vi "Random XY Generator.vi"(4 "Max h variatie":dbl=5.0, 5 "Max V variatie":dbl=1.0, 6 "Random Methode":u16(ring)=1 items=["Methode Random", "Methode smooth"], 7 "Y start":dbl=30.0, 8 "X start":dbl=61.0, 9 "number of rounds":i32=1) -> (0 "Array":cluster{"x":dbl, "y":dbl, "v":dbl, "h":dbl}[](array[cluster]), 1 "Array":dbl[][](array[numeric]), 2 "Y end randomized":dbl, 3 "X end randomized":dbl)   [LabVIEW 2014]
panel:
  out "XY Graph 2":cluster{dbl[], dbl[]}(graph)
  out "Y start 2":dbl
  out "X start 2":dbl
  out "Waveform Graph 2":dbl[](graph)
  out "Waveform Graph":dbl[](graph)
  out "XY Graph":cluster{dbl[], dbl[]}(graph)
  in  "Step Time [Sec]":dbl=1.0
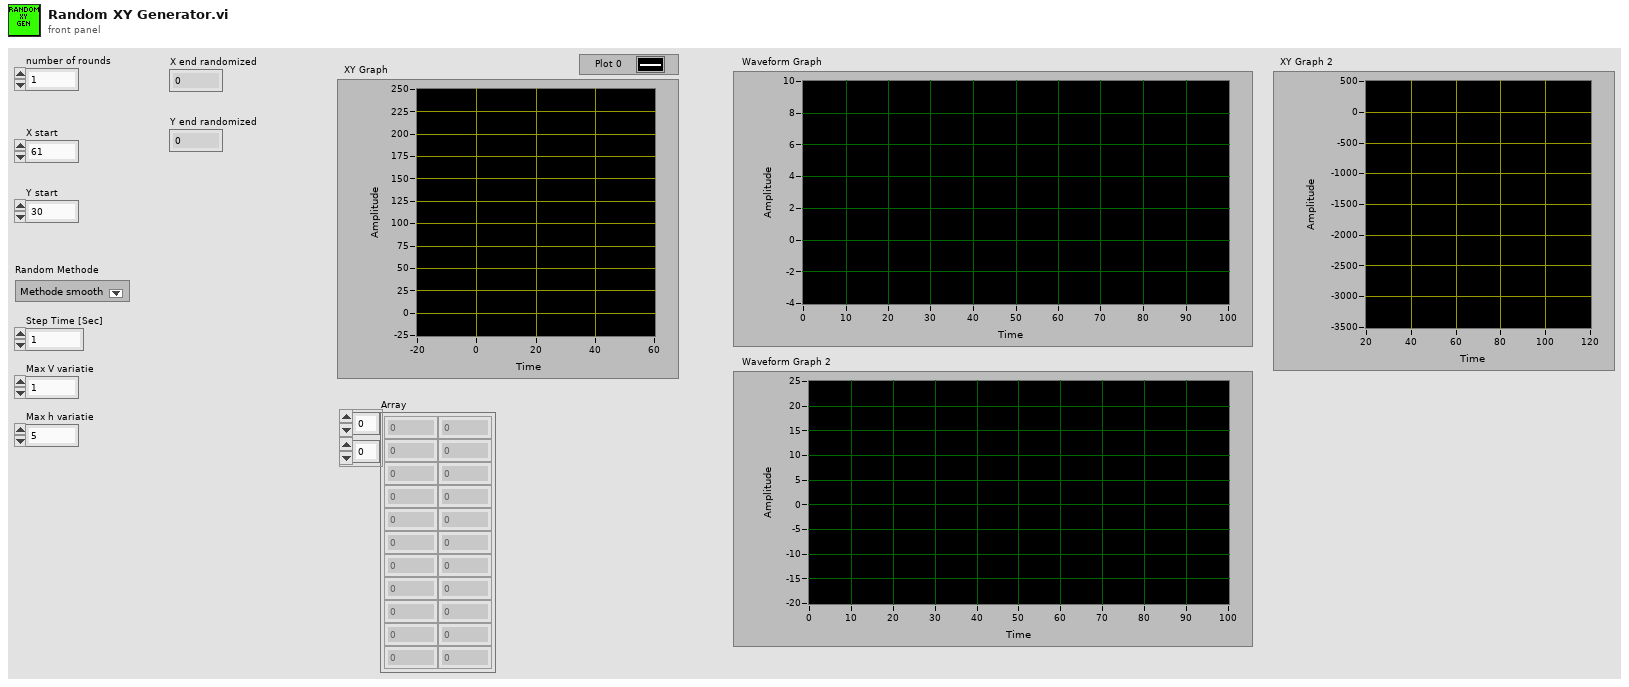
[diagram p1: front panel]
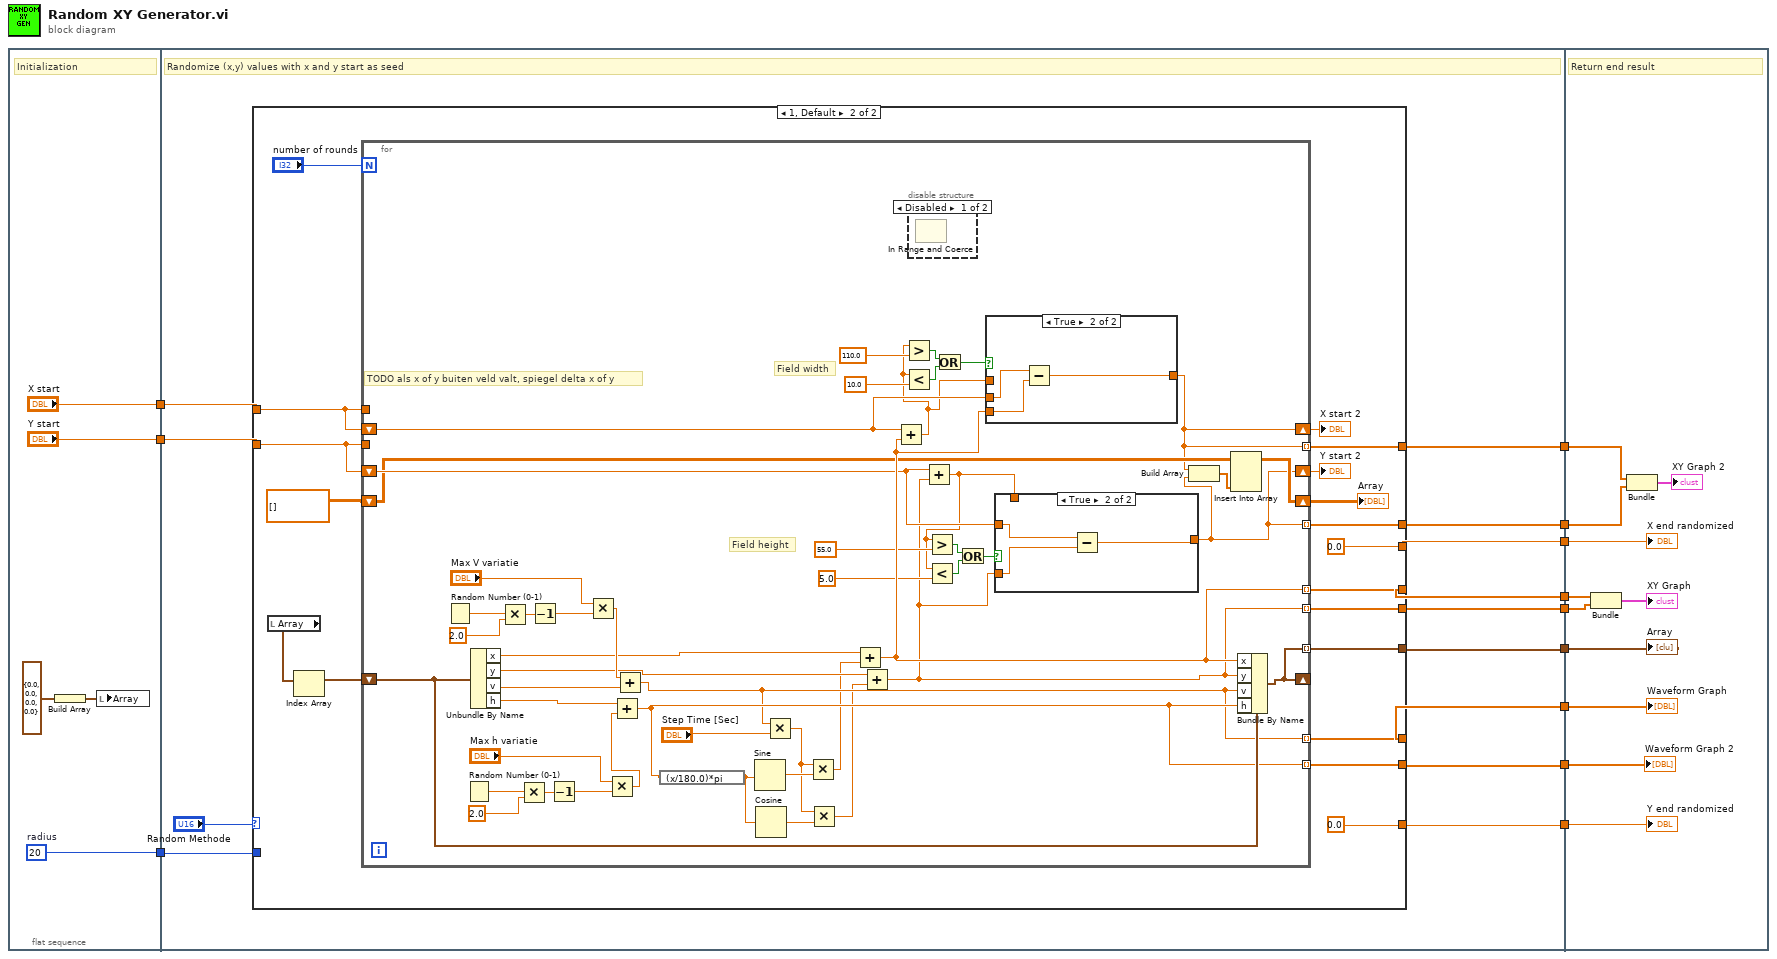
[diagram p0: block diagram]
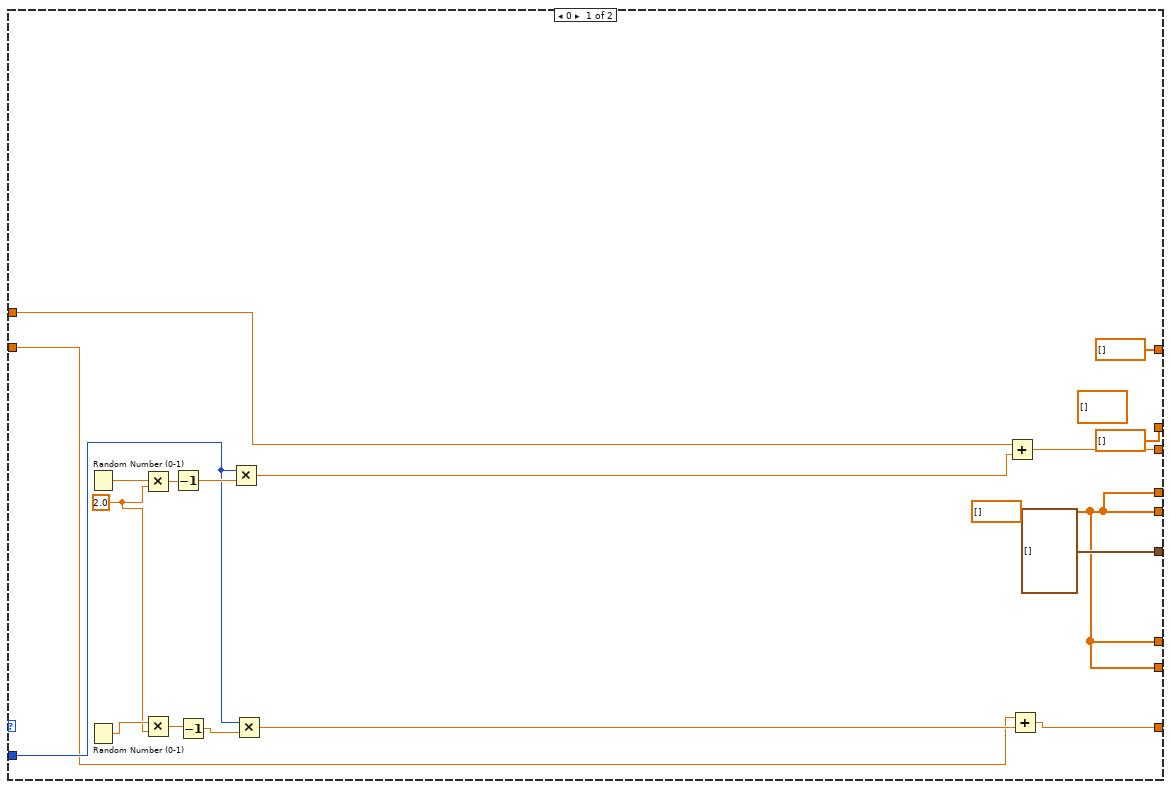
[diagram p2: hidden frame]
diagram:
  n1 = flat-sequence {
    tunnel: ["X start"] -> w12
    tunnel: ["Y start"] -> w11
    tunnel: [w15] -> w10
    tunnel: w12 -> [w29]
    tunnel: w11 -> [w28]
    tunnel: w10 -> [w30]
    tunnel: [w27] -> w9
    tunnel: [w26] -> w8
    tunnel: [w24] -> w7
    tunnel: [w23] -> w6
    tunnel: [w22] -> w5
    tunnel: [w21] -> w4
    tunnel: [w20] -> w3
    tunnel: [w19] -> w2
    tunnel: [w18] -> w1
    tunnel: w9 -> [w133]
    tunnel: w8 -> [w132]
    tunnel: w7 -> [w131]
    tunnel: w6 -> [w130]
    tunnel: w5 -> [w129]
    tunnel: w4 -> [w127]
    tunnel: w3 -> [w126]
    tunnel: w2 -> [w124]
    tunnel: w1 -> [w123]
    frame #0 {
      w15 = 20  # radius
      # "Initialization"
      n2 = Build Array(cluster{"x":dbl, "y":dbl, "v":dbl, "h":dbl} {"x"=0.0, "y"=0.0, "v"=0.0, "h"=0.0} ("Cluster")) -> (w13:cluster{"x":dbl, "y":dbl, "v":dbl, "h":dbl}[])
      n3 = local write "Array"(w13) -> ()
    }
    frame #1 {
      # "Randomize (x,y) values with x and y start as seed"
      n4 = case shown="1, Default" "Random Methode" {
        tunnel: w30 -> [w41 _]
        tunnel: w29 -> [w39 w57]
        tunnel: w28 -> [w37 w56]
        tunnel: [w36 0.0] -> w27
        tunnel: [w35 0.0] -> w26
        tunnel: [cluster{"x":dbl, "y":dbl, "v":dbl, "h":dbl}[] [] w66] -> w24
        tunnel: [w33 w63] -> w23
        tunnel: [w33 w62] -> w22
        tunnel: [w33 w59] -> w21
        tunnel: [w33 w58] -> w20
        tunnel: [dbl[] [] w51] -> w19
        tunnel: [dbl[] [] w50] -> w18
        frame 0 {
          (unwired) dbl[][] []
          w33 = dbl[] []
          w46 = 2.0
          n5 = Random Number (0-1)() -> (number: 0 to 1=w48:dbl)
          n6 = Random Number (0-1)() -> (number: 0 to 1=w47:dbl)
          n7 = Multiply(x=w48, y=w46) -> (x*y=w45:dbl)
          n8 = Multiply(x=w47, y=w46) -> (x*y=w44:dbl)
          n9 = Decrement(x=w45) -> (x-1=w43:dbl)
          n10 = Decrement(x=w44) -> (x-1=w42:dbl)
          n11 = Multiply(x=w41, y=w43) -> (x*y=w40:dbl)
          n12 = Multiply(x=w41, y=w42) -> (x*y=w38:dbl)
          n13 = Add(x=w39, y=w40) -> (x+y=w36:dbl)
          n14 = Add(x=w37, y=w38) -> (x+y=w35:dbl)
        }
        frame 1, Default {
          n15 = local read "Array"() -> (w61:cluster{"x":dbl, "y":dbl, "v":dbl, "h":dbl}[])
          n16 = Index Array(array=w61) -> (element=w60:cluster{"x":dbl, "y":dbl, "v":dbl, "h":dbl})  [unwired: 1 in]
          n17 = for {
            N: "number of rounds" -> [_]
            shift-right: [w97] -> _
            shift-left: w60 -> [w98]
            tunnel: [w97] -> w66 mode=indexing
            tunnel: [w81] -> w63 mode=indexing
            tunnel: [w74] -> w62 mode=indexing
            tunnel: [w92] -> w59 mode=indexing
            tunnel: [w93] -> w58 mode=indexing
            tunnel: w57 -> [_]
            tunnel: w56 -> [_]
            shift-right: [w68] -> w55
            shift-left: w57 -> [w82]
            shift-right: [w67] -> w54
            shift-left: w56 -> [w75]
            shift-right: [w71] -> w52
            shift-left: dbl[][] [] -> [w72]
            tunnel: [w68] -> w51 mode=indexing
            tunnel: [w67] -> w50 mode=indexing
            # "Field width"
            # "Field height"
            # "TODO als x of y buiten veld valt, spiegel delta x of y"
            n18 = Random Number (0-1)() -> (number: 0 to 1=w111:dbl)
            n19 = Random Number (0-1)() -> (number: 0 to 1=w107:dbl)
            n20 = Unbundle By Name(w98) -> ("x"=w91:dbl, "y"=w90:dbl, "v"=w96:dbl, "h"=w95:dbl)
            n21 = Multiply(x=w111, y=2.0) -> (x*y=w113:dbl)
            n22 = Multiply(x=w107, y=2.0) -> (x*y=w105:dbl)
            n23 = Decrement(x=w113) -> (x-1=w114:dbl)
            n24 = Decrement(x=w105) -> (x-1=w104:dbl)
            n25 = Multiply(x="Max V variatie", y=w114) -> (x*y=w109:dbl)
            n26 = Multiply(x="Max h variatie", y=w104) -> (x*y=w103:dbl)
            n27 = Add(x=w95, y=w103) -> (x+y=w93:dbl)
            n28 = Add(x=w109, y=w96) -> (x+y=w92:dbl)
            n29 = expression code="(x/180.0)*pi" ("degrees to radians")(w93) -> (w94:dbl)
            n30 = Sine(x=w94) -> (sin(x)=w101:dbl)
            n31 = Cosine(x=w94) -> (cos(x)=w102:dbl)
            n32 = Multiply(x=w92, y="Step Time [Sec]") -> (x*y=w100:dbl)
            n33 = Multiply(x=w100, y=w101) -> (x*y=w89:dbl)
            n34 = Multiply(x=w100, y=w102) -> (x*y=w88:dbl)
            n35 = Add(x=w91, y=w89) -> (x+y=w81:dbl)
            n36 = Add(x=w90, y=w88) -> (x+y=w74:dbl)
            n37 = Add(x=w82, y=w81) -> (x+y=w69:dbl)
            n38 = Greater?(x=w69, y=110.0) -> (0:w87:bool)
            n39 = Less?(x=w69, y=10.0) -> (x < y?=w86:bool)
            n40 = disable-structure shown="Disabled" {
              frame Disabled {
                n41 = In Range and Coerce() -> ()  [unwired: 3 in, 2 out]
              }
              frame Enabled {
              }
            }
            n42 = Add(x=w75, y=w74) -> (x+y=w73:dbl)
            n43 = Greater?(x=w73, y=55.0) -> (0:w79:bool)
            n44 = Less?(x=w73, y=5.0) -> (x < y?=w78:bool)
            n45 = Or(x=w87, y=w86) -> (x .or. y?=w85:bool)
            n46 = Or(x=w79, y=w78) -> (x .or. y?=w80:bool)
            n47 = case shown="True" w85 {
              tunnel: w82 -> [_ w122]
              tunnel: w81 -> [_ w121]
              tunnel: [w119 w120] -> w68
              tunnel: w69 -> [w119 _]
              frame False {
              }
              frame True {
                n48 = Subtract(x=w122, y=w121) -> (x-y=w120:dbl)
              }
            }
            n49 = case shown="True" w80 {
              tunnel: w73 -> [w115 _]
              tunnel: [w115 w118] -> w67
              tunnel: w75 -> [_ w117]
              tunnel: w74 -> [_ w116]
              frame False {
              }
              frame True {
                n50 = Subtract(x=w117, y=w116) -> (x-y=w118:dbl)
              }
            }
            n51 = Build Array(w68, w67) -> (w70:dbl[])
            n52 = Insert Into Array(array=w72, new element=w70) -> (w71:dbl[][])  [unwired: 2 in]
            n53 = Bundle By Name(cluster=w98, "x"=w81, "y"=w74, "v"=w92, "h"=w93) -> (w97:cluster{"x":dbl, "y":dbl, "v":dbl, "h":dbl})
          }
          "X start 2" <- w55
          "Y start 2" <- w54
          "Array" <- w52
        }
      }
    }
    frame #2 {
      # "Return end result"
      n54 = Bundle(w130, w129) -> (→"XY Graph":cluster{dbl[], dbl[]})  [unwired: 1 in]
      n55 = Bundle(w124, w123) -> (→"XY Graph 2":cluster{dbl[], dbl[]})  [unwired: 1 in]
      "X end randomized" <- w133
      "Y end randomized" <- w132
      "Array" <- w131
      "Waveform Graph" <- w127
      "Waveform Graph 2" <- w126
    }
  }
